vi "Read Attribute.vi"(10 "Attribute to Read":string, 11 "Object Attributes IN":string[][](array[string])) -> (1 "Found?":bool, 2 "Attribute Value":string, 3 "Object Attributes OUT":string[][](array[string]))   [LabVIEW 2017]
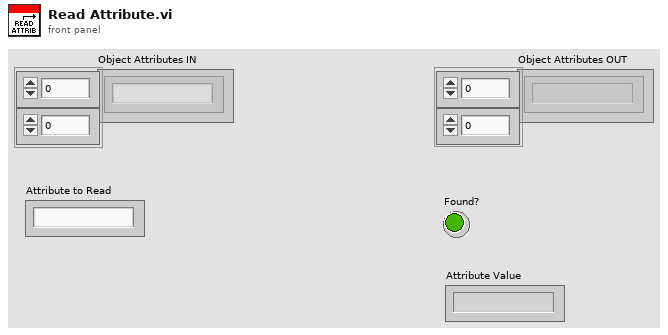
[diagram p1: front panel]
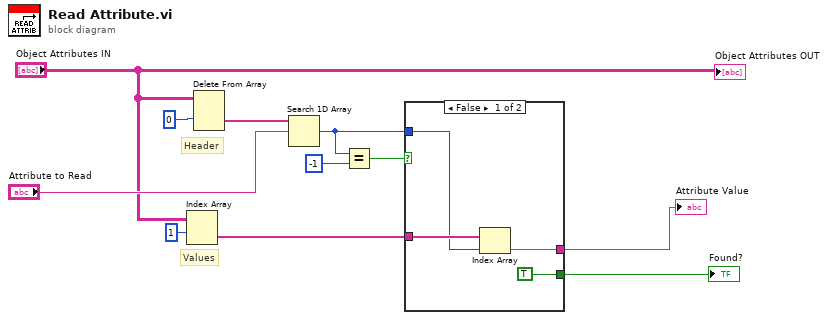
[diagram p0: block diagram]
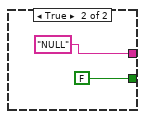
[diagram p2: hidden frame]
diagram:
  # "Values"
  # "Header"
  n1 = Index Array(array="Object Attributes IN", index (row)=1) -> (element=w9:string[])  [unwired: 1 in]
  n2 = Delete From Array(array="Object Attributes IN", index (row)=0) -> (deleted portion=w5:string[])  [unwired: 2 in, 1 out]
  n3 = Search 1D Array(1D array=w5, element="Attribute to Read") -> (index of element=w8:i32)  [unwired: 1 in]
  n4 = Equal?(x=w8, y=-1 ("index (row)")) -> (x = y?=w6:bool)
  n5 = case shown="False" w6 {
    tunnel: w9 -> [w15 _]
    tunnel: w8 -> [w14 _]
    tunnel: [TRUE FALSE] -> w3
    tunnel: [w12 "NULL"] -> w2
    frame False {
      n6 = Index Array(array=w15, index=w14) -> (element=w12:string)
    }
    frame True {
    }
  }
  "Attribute Value" <- w2
  "Found?" <- w3
  "Object Attributes OUT" <- "Object Attributes IN"
